vi "json_RemoveComment.vi"(1 "json with comment":string) -> (0 "json without comment":string)   [LabVIEW 2020]
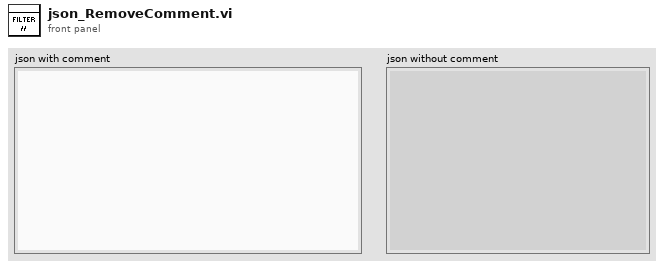
[diagram p1: front panel]
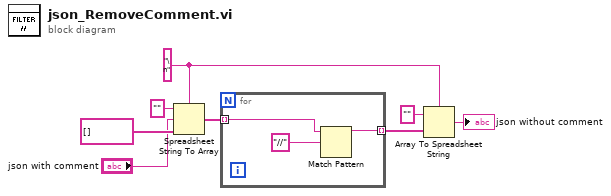
[diagram p0: block diagram]
diagram:
  w4 = "\n" ("delimiter (Tab)")
  n1 = Spreadsheet String To Array(delimiter (Tab)=w4, format string="", spreadsheet string="json with comment", array type (2D Dbl)=string[] []) -> (array=w6:string[])
  n2 = for {
    tunnel: w6 -> [w11] mode=indexing
    tunnel: [w9] -> w5 mode=indexing
    n3 = Match Pattern(string=w11, regular expression="//") -> (before substring=w9:string)  [unwired: 1 in, 3 out]
  }
  n4 = Array To Spreadsheet String(delimiter (Tab)=w4, array=w5, 3:"" ("format string")) -> (spreadsheet string=→"json without comment":string)
